vi "Accelerator_v2.001_small.vi"() -> ()   [LabVIEW 2013]
doc: "Acquire Accelerator Data"
uses:
  <instrlib>/niScope/Controls/niScope vertical coupling.ctl
  <instrlib>/niScope/Controls/niScope trigger slope.ctl
  <instrlib>/niScope/Controls/niScope trigger coupling.ctl
  <instrlib>/niScope/Controls/niScope trigger source.ctl
  Accelerator Measurement/Array_Defctl.ctl
  <vilib>/Utility/error.llb/DialogType.ctl
  <vilib>/Utility/miscctls.llb/LVPointTypeDef.ctl
  Public API/Dust_Event.ctl
  Public API/Signal.ctl
  Private/Role ID.ctl
  Private/Hardware ID.ctl
  Private/Estimate_source.ctl
  Functional Global Variables/Action Items.ctl
  <vilib>/Analysis/baseanly.llb/Mean (DBL).vi
  Private/PSU updated.vi
  <vilib>/addons/database/Connection.llb/Conn Execute.vi
  <vilib>/addons/database/Recordset.llb/Rec Fetch Recordset Data (R).vi
  <vilib>/addons/database/Recordset.llb/Rec Destroy - Connection.vi
  <instrlib>/niScope/Configure/Trigger/niScope Configure Trigger Edge.vi
  <instrlib>/niScope/Configure/Trigger/niScope Configure Trigger Immediate.vi
  <instrlib>/niScope/Acquire/Fetch/niScope Multi Fetch Cluster.vi
  <vilib>/addons/database/_DB Variant To Data/Database Variant To Data.xnode
  <vilib>/Analysis/NI_AALBase.lvlib
  <vilib>/addons/database/NI_Database_API.lvlib
panel:
  in  "Big Accelerator?":bool
  in  "Trigger":enum32{"Immediate", "Edge"}(tab)=enum."Edge"
  in  "Trigger Source Edge 2":T1="2" caption="Source"
  in  "Trigger Source Edge":T1="0" caption="Source"
  in  "Coupling":T2=1 items=["AC"=0, "DC"=1, "HF Reject"=3, "LF Reject"=4, "AC Plus HF Reject"=1001]
  in  "Slope":T3 caption="Trigger Slope"
  in  "Level":dbl=1.0 caption="Trigger Level" step=0.001 format="%.3f"
  in  "Delay":dbl caption="Trigger Delay" format="%.4p"
  in  "Reference Position (%)":dbl=40.0 caption="Ref Position" format="%.1f"
  in  "Bandwidth":dbl=-1.0 format="%.2f"
  in  "Vertical Coupling":T4=1 items=["AC", "DC", "Ground"]
  in  "Probe Attenuation":dbl=1.0 format="%.1f"
  in  "Vertical Offset":dbl format="%.4f"
  in  "Vertical Range":dbl=5.0 caption="Vertical Range (V)" format="%.2f"
  out "Actual Sample Rate":dbl=10000000.0 format="%.0p"
  in  "Min Record Length":i32=100000 caption="Min. Record Length"
  in  "Min Sample Rate":dbl=80000000.0 caption="Min. Sample Rate" step=1000000.0 format="%.2p"
  out "Actual Record Length":i32=100000
  out "Mass":dbl format="%#_3g"
  in  "Write to Database?":bool=TRUE
  in  "Limit":dbl
  in  "Limit Triggers":bool
  out "Acquisition #":i32
  in  "WFM Tag":string="trace"
  in  "Location":string="G:\\default"
  in  "Write Raw File?":bool
  out "Saving Raw File...":path=path "G:/2012_06_13_verify_timestamp_labview/trace00000"
  out "?":cluster{dbl, dbl}(knob)={0.0549, 2.0} scale=10.0..0.01
  in  "Ideal Time (Cursor)":dbl=2.0 step=0.01 format="%_2f"
  out "Time Between Triggers":dbl
  out "Average Frequency":dbl format="%#_4g"
  out "output cluster":T5
  out "error out 4":errorcluster
  out "error out 3":errorcluster
  out "# elements in queue":i32
  out "Stop condition":bool=TRUE
  out "created path":path=path "G:/default"
  out "Numeric":i32=92364
  out "error out 2":errorcluster
  out "Calibration":dbl=24700000000000.0
  out "Array":T6=["Dev1", "Dev2"]
  in  "Debug Mode\n(Confusing)":bool
  out "Multi Plot 2":cluster{dbl[], dbl[]}(graph) caption="Multi Plot"
  in  "Acceleration Voltage (MV)":dbl=2.0 format="%_2g"
  out "Charge":dbl format="%#_3g"
  out "Velocity (Est.)":dbl format="%#_6f"
  out "Final Detector (CH3)":waveform(dbl)(graph)={"t0"=timestamp(0 s since 1904-01-01), "dt"=1e-07, "Y"=[]}
  out "Charge Detector/PSU gate (CH2)":waveform(dbl)(graph)={"t0"=timestamp(0 s since 1904-01-01), "dt"=1e-07, "Y"=[]}
  out "Velocity Detectors (CH0 & CH1)":waveform(dbl)[](graph)
  in  "stop":bool=TRUE
  out "error out":errorcluster={"status"=FALSE, "code"=0, "source"="No Error"} {"code" format="%.0x"}
  # "File Parameters"
  # "Error Handling"
  # "Trigger"
  # "Channel"
  # "Vertical"
  # "Horizontal"
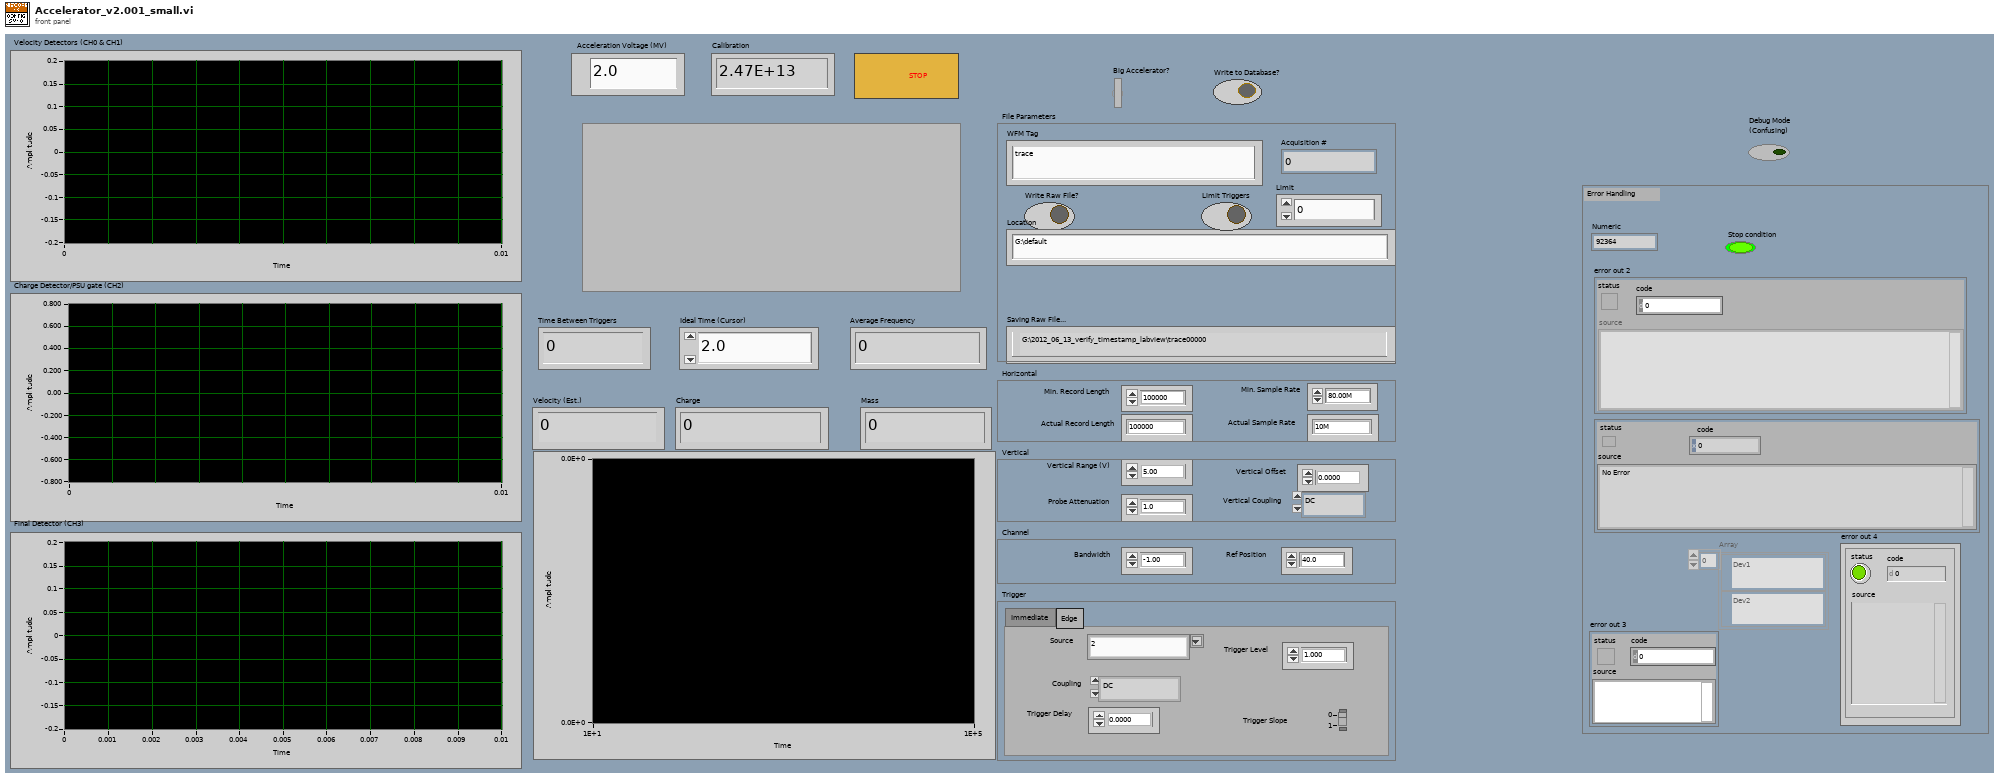
[diagram p1: front panel]
types:
  T1 = typedef "niScope trigger source.ctl" = string
  T2 = typedef "niScope trigger coupling.ctl" = u16
  T3 = typedef "niScope trigger slope.ctl" = i32
  T4 = typedef "niScope vertical coupling.ctl" = i32
  T5 = cluster{"File Path Control":path, "Array":waveform(dbl)[]}
  T6 = typedef "Array_Defctl.ctl" = refnum<k15>[]
  T7 = typedef "LVPointTypeDef.ctl" = cluster{"Horizontal":i16, "Vertical":i16}
  T8 = typedef "DialogType.ctl" = u16
  T9 = typedef "NI_Database_API.lvlib/Conn ObjectReference.ctl" = refnum<k1>
  T10 = typedef "NI_Database_API.lvlib/Rec ObjectReference.ctl" = refnum<k1>
  T11 = cluster{"Integer Timestamp":dbl, "Max Velocity":dbl, "Min Velocity":dbl}
  T12 = cluster{"first point time":dbl, "xIncrement":dbl, "Waveforms":dbl[]}[]
  T13 = typedef "Dust_Event.ctl" = cluster{"Time Stamp":timestamp, "Velocity":sgl, "Mass":sgl, "Charge":sgl, "Radius":sgl, "Array":T14[], "Dust Event ID":i64, "Passed_3rd_Detector":bool, "Estimate Source":T17, "Estimate Quality":sgl}
  T14 = typedef "Signal.ctl" = cluster{"Signal ID":i64, "Time Stamp":timestamp, "Dust Event ID":i64, "Role ID":T15, "Data":sgl[], "Signal Length":i32, "dt":sgl, "Offset":dbl, "Hardware ID":T16}
  T15 = typedef "Role ID.ctl" = enum16{"First_Detector", "Second_Detector", "Third_Detector", "LeCroy_CH1", "LeCroy_CH2", "LeCroy_CH3", "LeCroy_CH4", "PSU"}
  T16 = typedef "Hardware ID.ctl" = enum16{"Unknown", "CSA 1", "CSA 2", "CSA 3", "CSA 4", "CSA 5", "CSA 6"}
  T17 = typedef "Estimate_source.ctl" = i8
  T18 = typedef "Action Items.ctl" = enum16{"Initialize", "Get", "Set"}
  T19 = cluster{"relativeInitialX":dbl, "xIncrement":dbl, "wfm":dbl[]}[]
  T20 = cluster{"first point time":dbl, "xIncrement":dbl, "Waveforms":dbl[]}
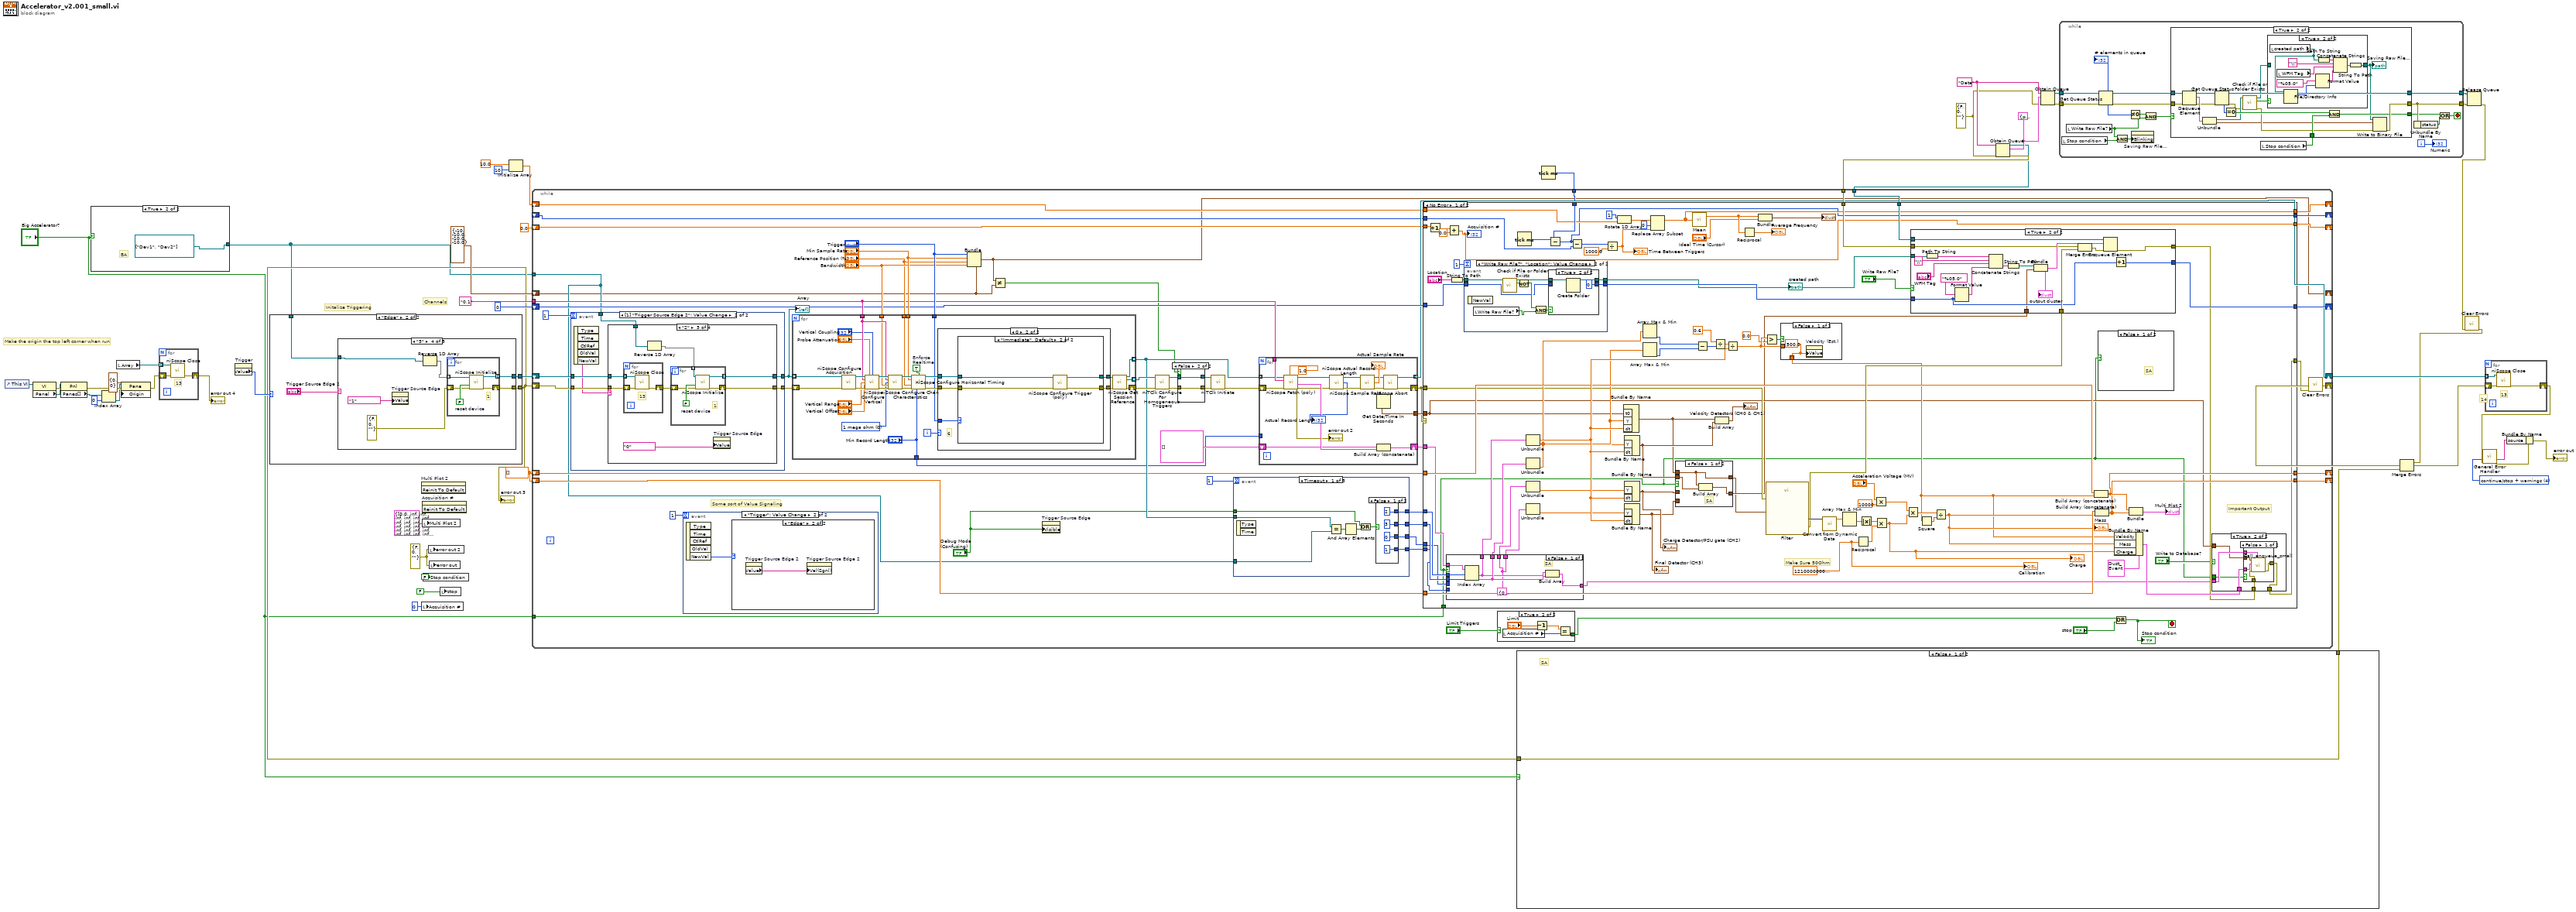
[diagram p0: block diagram]
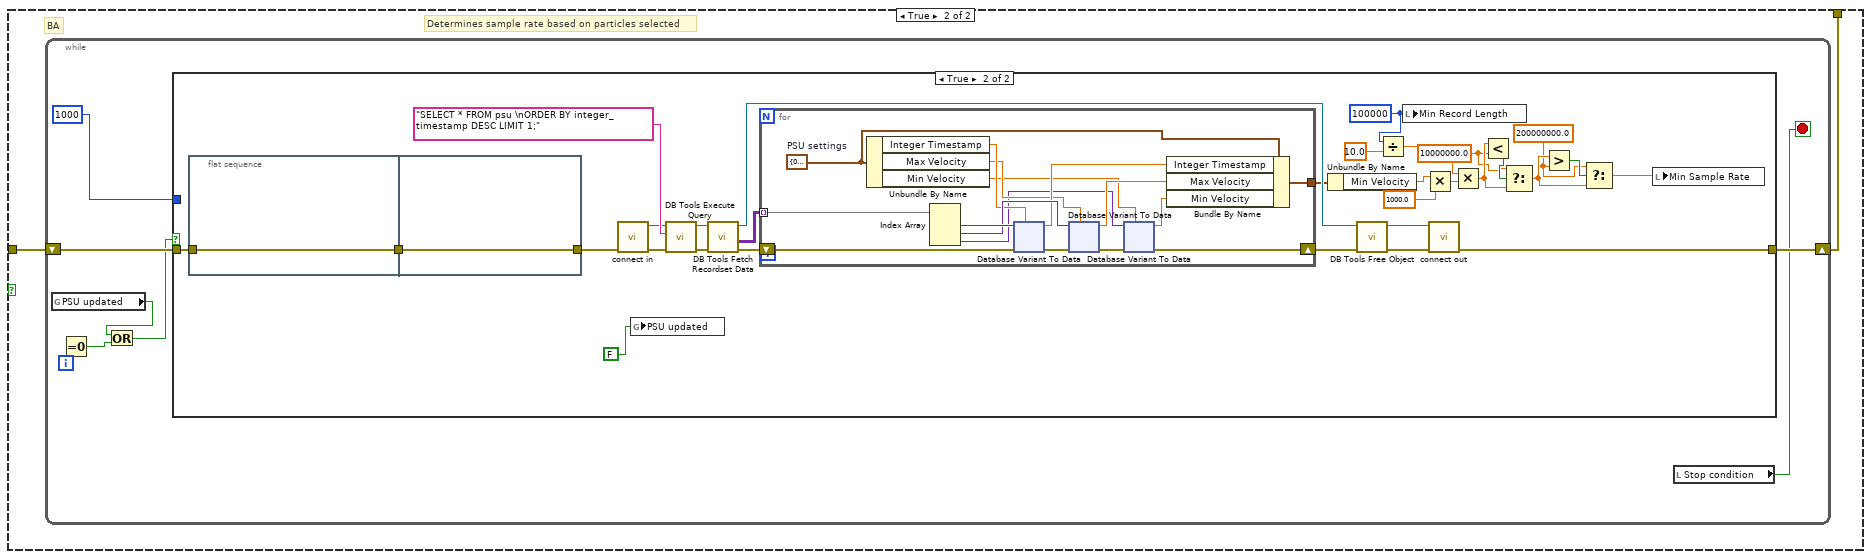
[diagram p2: hidden frame]
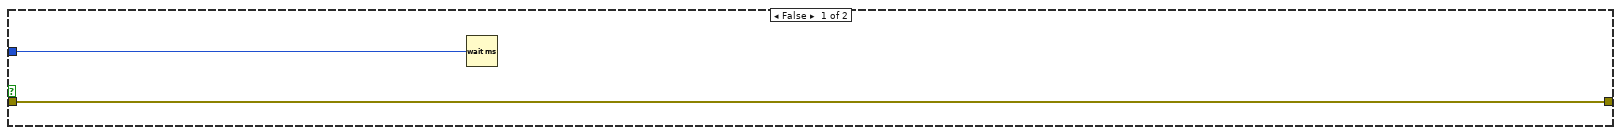
[diagram p3: hidden frame]
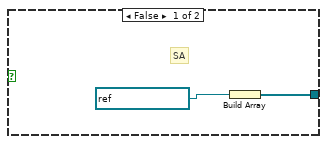
[diagram p4: hidden frame]
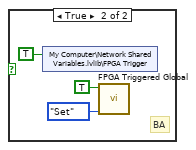
[diagram p5: hidden frame]
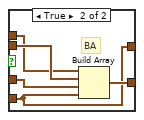
[diagram p6: hidden frame]
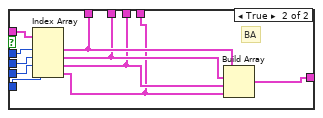
[diagram p7: hidden frame]
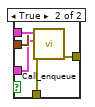
[diagram p9: hidden frame]
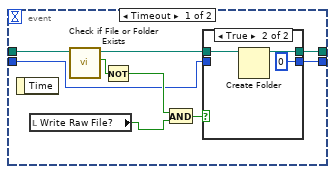
[diagram p10: hidden frame]
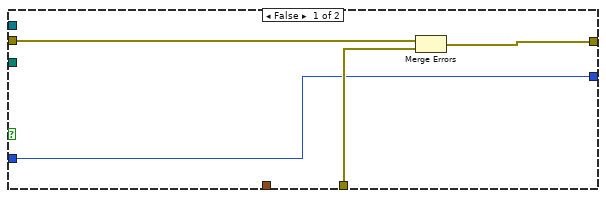
[diagram p13: hidden frame]
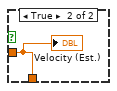
[diagram p14: hidden frame]
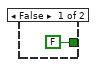
[diagram p16: hidden frame]
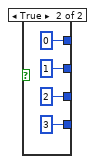
[diagram p17: hidden frame]
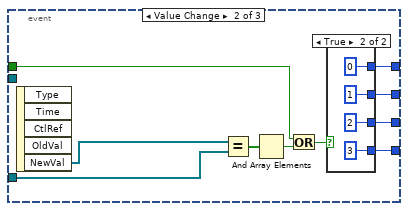
[diagram p18: hidden frame]
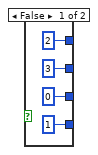
[diagram p19: hidden frame]
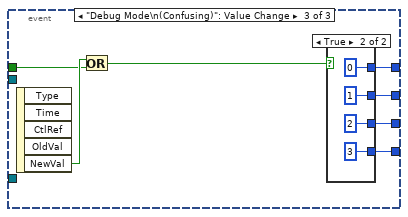
[diagram p20: hidden frame]
diagram:
  w15 = dbl[] []
  w22 = errorcluster {"status"=FALSE, "code"=0, "source"=""} ("error out")
  w27 = errorcluster {"status"=FALSE, "code"=0, "source"=""} ("error out")
  w28 = cluster{path, waveform(sgl)[]} {path "", []} ("output cluster")
  w29 = "Data" ("name (unnamed)")
  w20 = T8 4 items=["no dialog", "OK message", "continue or stop message", "OK message + warnings", "continue/stop + warnings"] ("type of dialog (OK msg:1)")
  # "Channels"
  # "Make the origin the top left corner when run"
  # "Initalize Triggering"
  # "14"
  n1 = control-ref of="This VI"() -> (w11:refnum<vi>)
  n2 = property class="VI"(reference=w11) -> (error out=w10:errorcluster, "Panel"=w9:refnum<vi>)  [unwired: 1 in, 1 out]
  n3 = property class="Pnl"(reference=w9, error in=w10) -> (error out=w8:errorcluster, "Panes[]"=w7:refnum<vi>[])  [unwired: 1 out]
  n4 = case shown="True" "Big Accelerator?" {
    tunnel: [w51 refnum<k15>[] ["Dev1", "Dev2"] ("Resources")] -> w2
    frame False {
      # "SA"
      n5 = Build Array(refnum<k15> "Dev1" ("resource name")) -> (w51:refnum<k15>[])
    }
    frame True {
      # "BA"
    }
  }
  n6 = Index Array(array=w7, index=0) -> (element=w5:refnum<vi>)
  n7 = local read "Array"() -> (w30:T6)
  n8 = property class="Pane"(reference=w5, error in=w8, "Origin"=T7 {"Horizontal"=0, "Vertical"=0}) -> (error out=w3:errorcluster)  [unwired: 1 out]
  n9 = for {
    tunnel: w30 -> [w54] mode=indexing
    shift-right: [w56] -> w25
    shift-left: w3 -> [w55]
    # "13"
    n10 = call <instrlib>:"niScope Close.vi"("instrument handle"=w54, "error in"=w55) -> ("error out"=w56:errorcluster)  [unwired: 13 in]
  }
  "error out 4" <- w25
  n11 = property on="Trigger" class="TabCtl (strict)"() -> ("Value"=w39:enum32{"Immediate", "Edge"})  [unwired: 2 in, 2 out]
  n12 = case shown="\"Edge\"" w39 {
    tunnel: [w59 w69] -> w49
    tunnel: [w58 w68] -> w13
    tunnel: w2 -> [w57 w66]
    frame "Immediate", Default {
      n13 = for {
        tunnel: w57 -> [w64] mode=indexing
        tunnel: [w62] -> w59 mode=indexing
        shift-right: [w61] -> w58
        shift-left: errorcluster {"status"=FALSE, "code"=0, "source"=""} ("error out") -> [w63]
        w65 = FALSE  # reset device
        n14 = call <instrlib>:"niScope Initialize.vi"("resource name"=w64, "reset device"=w65, "error in"=w63) -> ("instrument handle"=w62:refnum<k15>, "error out"=w61:errorcluster)  [unwired: 11 in]
      }
    }
    frame "Edge" {
      n15 = case shown="\"3\"" "Trigger Source Edge 2" {
        tunnel: [w74 w83 w94 w105 w116] -> w69
        tunnel: [w73 w82 w93 w104 w115] -> w68
        tunnel: w66 -> [w70 w80 w90 w101 w112]
        frame "0", Default {
          n16 = property on="Trigger Source Edge" class="CmbBox (strict)"("Value"=T1 "0" ("Trigger Source Edge")) -> ()  [unwired: 2 in, 2 out]
          n17 = for {
            tunnel: w70 -> [w78] mode=indexing
            tunnel: [w76] -> w74 mode=indexing
            shift-right: [w75] -> w73
            shift-left: errorcluster {"status"=FALSE, "code"=0, "source"=""} ("error out") -> [w77]
            w79 = FALSE  # reset device
            n18 = call <instrlib>:"niScope Initialize.vi"("resource name"=w78, "reset device"=w79, "error in"=w77) -> ("instrument handle"=w76:refnum<k15>, "error out"=w75:errorcluster)  [unwired: 11 in]
          }
        }
        frame "1" {
          n19 = property on="Trigger Source Edge" class="CmbBox (strict)"("Value"=T1 "1" ("Trigger Source Edge")) -> ()  [unwired: 2 in, 2 out]
          n20 = for {
            tunnel: w80 -> [w88] mode=indexing
            tunnel: [w86] -> w83 mode=indexing
            shift-right: [w85] -> w82
            shift-left: errorcluster {"status"=FALSE, "code"=0, "source"=""} ("error out") -> [w87]
            w89 = FALSE  # reset device
            # "1"
            n21 = call <instrlib>:"niScope Initialize.vi"("resource name"=w88, "reset device"=w89, "error in"=w87) -> ("instrument handle"=w86:refnum<k15>, "error out"=w85:errorcluster)  [unwired: 11 in]
          }
        }
        frame "2" {
          n22 = property on="Trigger Source Edge" class="CmbBox (strict)"("Value"=T1 "0" ("Trigger Source Edge")) -> ()  [unwired: 2 in, 2 out]
          n23 = Reverse 1D Array(array=w90) -> (reversed array=w91:refnum<k15>[])
          n24 = for {
            tunnel: w91 -> [w99] mode=indexing
            tunnel: [w97] -> w94 mode=indexing
            shift-right: [w96] -> w93
            shift-left: errorcluster {"status"=FALSE, "code"=0, "source"=""} ("error out") -> [w98]
            w100 = FALSE  # reset device
            # "1"
            n25 = call <instrlib>:"niScope Initialize.vi"("resource name"=w99, "reset device"=w100, "error in"=w98) -> ("instrument handle"=w97:refnum<k15>, "error out"=w96:errorcluster)  [unwired: 11 in]
          }
        }
        frame "3" {
          n26 = property on="Trigger Source Edge" class="CmbBox (strict)"("Value"=T1 "1" ("Trigger Source Edge")) -> ()  [unwired: 2 in, 2 out]
          n27 = Reverse 1D Array(array=w101) -> (reversed array=w102:refnum<k15>[])
          n28 = for {
            tunnel: w102 -> [w110] mode=indexing
            tunnel: [w108] -> w105 mode=indexing
            shift-right: [w107] -> w104
            shift-left: errorcluster {"status"=FALSE, "code"=0, "source"=""} ("error out") -> [w109]
            w111 = FALSE  # reset device
            # "1"
            n29 = call <instrlib>:"niScope Initialize.vi"("resource name"=w110, "reset device"=w111, "error in"=w109) -> ("instrument handle"=w108:refnum<k15>, "error out"=w107:errorcluster)  [unwired: 11 in]
          }
        }
        frame "VAL_EXTERNAL" {
          n30 = property on="Trigger Source Edge" class="CmbBox (strict)"("Value"=T1 "VAL_EXTERNAL" ("Trigger Source Edge")) -> ()  [unwired: 2 in, 2 out]
          n31 = for {
            tunnel: w112 -> [w120] mode=indexing
            tunnel: [w118] -> w116 mode=indexing
            shift-right: [w117] -> w115
            shift-left: errorcluster {"status"=FALSE, "code"=0, "source"=""} ("error out") -> [w119]
            w121 = FALSE  # reset device
            n32 = call <instrlib>:"niScope Initialize.vi"("resource name"=w120, "reset device"=w121, "error in"=w119) -> ("instrument handle"=w118:refnum<k15>, "error out"=w117:errorcluster)  [unwired: 11 in]
          }
        }
      }
    }
  }
  "error out 3" <- w13
  n33 = invoke on="Multi Plot 2" class="XYGraph (strict)" method="Reinit To Default"() -> ()  [unwired: 3 in, 3 out]
  n34 = local write "Acquisition #"(0 ("Acquisition #")) -> ()
  n35 = invoke on="Acquisition #" class="DigNum (strict)" method="Reinit To Default"() -> ()  [unwired: 3 in, 3 out]
  n36 = local write "Multi Plot 2"(cluster{dbl[], dbl[]} {[0.0, inf, inf, inf, inf, inf, inf, inf, inf, inf, inf, inf, inf, inf, inf, inf, inf, inf, inf, inf, inf, inf, inf, inf, inf, inf, inf, inf, inf, inf, inf, inf, inf, inf, inf, inf, inf, inf, inf, inf, inf], [0.0, 0.0, 0.0, 0.0, 0.0, 0.0, 0.0, 0.0, 0.0, 0.0, 0.0, 0.0, 0.0, 0.0, 0.0, 0.0, 0.0, 0.0, 0.0, 0.0, 0.0, 0.0, 0.0, 0.0, 0.0, 0.0, 0.0, 0.0, 0.0, 0.0, 0.0, 0.0, 0.0, 0.0, 0.0, 0.0, 0.0, 0.0, 0.0, 0.0, 0.0]} ("Multi Plot 2")) -> ()
  n37 = local write "Stop condition"(FALSE ("x .or. y?")) -> ()
  n38 = local write "error out 2"(w22) -> ()
  n39 = local write "error out"(w22) -> ()
  n40 = local write "stop"(FALSE ("stop")) -> ()
  n41 = Initialize Array(10.0 ("element"), 10 ("dimension size")) -> (w41:dbl[])
  n42 = case shown="False" "Big Accelerator?" {
    tunnel: w13 -> [w122 w124]
    tunnel: [w122 w123] -> w12
    frame False {
      # "SA"
    }
    frame True {
      # "BA"
      # "Determines sample rate based on particles selected"
      n43 = while {
        shift-right: [w131] -> w123
        shift-left: w124 -> [w132]
        i -> [w130]
        stop <- w129 stop-if-true
        n44 = global read "PSU updated.vi" "PSU updated"() -> (w128:bool)
        n45 = Equal To 0?(x=w130) -> (x = 0?=w126:bool)
        n46 = Or(x=w128, y=w126) -> (x .or. y?=w127:bool)
        n47 = case shown="True" w127 {
          tunnel: w132 -> [w133 w163]
          tunnel: [w133 w162] -> w131
          tunnel: 1000 -> [w134 _]
          frame False {
            n48 = Wait (ms)(milliseconds to wait=w134) -> ()  [unwired: 1 out]
          }
          frame True {
            w136 = 200000000.0 ("y")
            w139 = 10000000.0 ("y")
            w146 = 100000 ("Min Record Length")
            n49 = flat-sequence {
              tunnel: [w165] -> w164
              tunnel: w163 -> [w165]
              tunnel: w164 -> [w166]
              tunnel: [w166] -> w149
              frame #0 {
              }
              frame #1 {
              }
            }
            n50 = call "connect in.vi"("error in (no error)"=w149) -> ("error out"=w153:errorcluster, "Database Connection"=w152:T9)  [unwired: 6 in, 1 out]
            n51 = global write "PSU updated.vi" "PSU updated"(FALSE ("PSU updated")) -> ()
            n52 = call-poly <vilib>:"DB Tools Execute Query.vi"("error in (no error)"=w153, "SQL query"="SELECT * FROM psu \nORDER BY integer_timestamp DESC LIMIT 1;", "connection reference"=w152) -> ("error out"=w155:errorcluster, "recordset reference"=w154:T10)  [unwired: 5 in]
            n53 = call-poly <vilib>:"DB Tools Fetch Recordset Data.vi"("error in (no error)"=w155, "recordset reference"=w154) -> ("error out"=w161:errorcluster, "recordset data"=w160:variant[][], "recordset reference out"=w156:T10)  [unwired: 3 in]
            n54 = for {
              tunnel: w160 -> [w182] mode=indexing
              shift-right: [w167] -> w150
              shift-left: w161 -> [w178]
              tunnel: [w177] -> w151
              w172 = T11 {"Integer Timestamp"=0.0, "Max Velocity"=0.0, "Min Velocity"=0.0}  # PSU settings
              n55 = Unbundle By Name(w172) -> ("Integer Timestamp"=w176:dbl, "Max Velocity"=w173:dbl, "Min Velocity"=w170:dbl)
              n56 = Index Array(array=w182) -> (element #1=w181:variant, element #2=w180:variant, element #3=w171:variant)  [unwired: 3 in]
              n57 = xnode "Database Variant To Data"("database variant"=w181, "error in"=w178, "type"=w176) -> ("data"=w175:dbl, "error out"=w179:errorcluster)
              n58 = xnode "Database Variant To Data"("database variant"=w180, "error in"=w179, "type"=w173) -> ("data"=w174:dbl, "error out"=w168:errorcluster)
              n59 = xnode "Database Variant To Data"("database variant"=w171, "error in"=w168, "type"=w170) -> ("data"=w169:dbl, "error out"=w167:errorcluster)
              n60 = Bundle By Name(cluster=w172, "Integer Timestamp"=w175, "Max Velocity"=w174, "Min Velocity"=w169) -> (w177:T11)
            }
            n61 = Unbundle By Name(w151) -> ("Min Velocity"=w145:dbl)
            n62 = call-poly <vilib>:"DB Tools Free Object.vi"("error in (no error)"=w150, "recordset reference"=w156) -> ("error out"=w157:errorcluster, "connection reference"=w158:T9)  [unwired: 8 in]
            n63 = Divide(x=w146, y=10.0) -> (x/y=w142:dbl)
            n64 = local write "Min Record Length"(w146) -> ()
            n65 = Multiply(x=w145, y=1000.0) -> (x*y=w143:dbl)
            n66 = call "connect out.vi"("error in (no error)"=w157, "connection reference"=w158) -> ("error out"=w162:errorcluster)  [unwired: 9 in]
            n67 = Multiply(x=w142, y=w143) -> (x*y=w140:dbl)
            n68 = Less?(x=w140, y=w139) -> (x < y?=w141:bool)
            n69 = Select(t=w139, s=w141, f=w140) -> (s? t:f=w138:dbl)
            n70 = Greater?(x=w138, y=w136) -> (0:w137:bool)
            n71 = Select(t=w136, s=w137, f=w138) -> (s? t:f=w135:dbl)
            n72 = local write "Min Sample Rate"(w135) -> ()
          }
        }
        n73 = local read "Stop condition"() -> (w129:bool)
      }
    }
  }
  n74 = Tick Count (ms)() -> (millisecond timer value=w44:u32)
  n75 = Obtain Queue(name (unnamed)=w29, element data type=w28, error in (no error)=w27) -> (queue out=w24:refnum<queue>, error out=w37:errorcluster)  [unwired: 2 in, 1 out]
  n76 = while {
    shift-right: [w291] -> w23
    shift-left: w13 -> [w296]
    shift-right: [w280] -> _
    shift-left: cluster{i32, dbl, dbl, dbl} {-10, -10.0, -10.0, -10.0} -> [w281]
    tunnel: w44 -> [w288]
    shift-right: [w286] -> _
    shift-left: w41 -> [w287]
    shift-right: [w285] -> _
    shift-left: _ -> [w289]
    shift-right: [w323] -> _
    shift-left: w15 -> [w300]
    shift-right: [w322] -> _
    shift-left: w15 -> [w321]
    tunnel: "0,1" ("Channel Name") -> [w320]
    shift-right: [w297] -> w38
    shift-left: w49 -> [w318]
    tunnel: w24 -> [w307]
    tunnel: w37 -> [w306]
    shift-right: [w305] -> _
    shift-left: 0 -> [w304]
    shift-right: [w283] -> _
    shift-left: 0.0 -> [w284]
    tunnel: w2 -> [w282]
    tunnel: "Big Accelerator?" -> [w279]
    stop <- w295 stop-if-true
    # "Some sort of Value Signaling"
    n77 = event shown="[1] \"Trigger Source Edge 2\": Value Change" {
      selector: _ -> [_ _]
      dyn-events: _ -> [_ _]
      timeout: 1 -> [_ _]
      tunnel: w318 -> [w604 w609]
      tunnel: [w604 w607] -> w315
      tunnel: w296 -> [w603 w610]
      tunnel: [w603 w606] -> w316
      tunnel: w282 -> [_ w605]
      event Timeout {
        n78 = event-data() -> ()  [unwired: 1 in, 2 out]
      }
      event Value Change {
        n79 = event-data() -> ("NewVal"=w608:T1)  [unwired: 1 in, 4 out]
        n80 = case shown="\"2\"" w608 {
          selector: w608 -> [w612 w627 _ _]
          tunnel: w609 -> [w614 w629 w647 w661]
          tunnel: [w616 w631 w645 w662] -> w607
          tunnel: w610 -> [w613 w628 w646 w660]
          tunnel: [w615 w630 w644 w663] -> w606
          tunnel: w605 -> [w611 w626 w641 w658]
          frame "0", Default {
            n81 = for {
              tunnel: w614 -> [w618] mode=indexing
              shift-right: [w620] -> w617
              shift-left: w613 -> [w619]
              # "13"
              n82 = call <instrlib>:"niScope Close.vi"("instrument handle"=w618, "error in"=w619) -> ("error out"=w620:errorcluster)  [unwired: 13 in]
            }
            n83 = for {
              tunnel: [w624] -> w616 mode=indexing
              shift-right: [w623] -> w615
              shift-left: w617 -> [w621]
              tunnel: w611 -> [w622] mode=indexing
              w625 = FALSE  # reset device
              # "1"
              n84 = call <instrlib>:"niScope Initialize.vi"("resource name"=w622, "reset device"=w625, "error in"=w621) -> ("instrument handle"=w624:refnum<k15>, "error out"=w623:errorcluster)  [unwired: 11 in]
            }
            n85 = property on="Trigger Source Edge" class="CmbBox (strict)"("Value"=w612) -> ()  [unwired: 2 in, 2 out]
          }
          frame "1" {
            n86 = for {
              tunnel: w629 -> [w633] mode=indexing
              shift-right: [w635] -> w632
              shift-left: w628 -> [w634]
              # "13"
              n87 = call <instrlib>:"niScope Close.vi"("instrument handle"=w633, "error in"=w634) -> ("error out"=w635:errorcluster)  [unwired: 13 in]
            }
            n88 = for {
              tunnel: [w639] -> w631 mode=indexing
              shift-right: [w638] -> w630
              shift-left: w632 -> [w636]
              tunnel: w626 -> [w637] mode=indexing
              w640 = FALSE  # reset device
              # "1"
              n89 = call <instrlib>:"niScope Initialize.vi"("resource name"=w637, "reset device"=w640, "error in"=w636) -> ("instrument handle"=w639:refnum<k15>, "error out"=w638:errorcluster)  [unwired: 11 in]
            }
            n90 = property on="Trigger Source Edge" class="CmbBox (strict)"("Value"=w627) -> ()  [unwired: 2 in, 2 out]
          }
          frame "2" {
            n91 = for {
              tunnel: w647 -> [w649] mode=indexing
              shift-right: [w651] -> w648
              shift-left: w646 -> [w650]
              # "13"
              n92 = call <instrlib>:"niScope Close.vi"("instrument handle"=w649, "error in"=w650) -> ("error out"=w651:errorcluster)  [unwired: 13 in]
            }
            n93 = Reverse 1D Array(array=w641) -> (reversed array=w642:refnum<k15>[])
            n94 = for {
              tunnel: [w655] -> w645 mode=indexing
              shift-right: [w654] -> w644
              shift-left: w648 -> [w652]
              tunnel: w642 -> [w653] mode=indexing
              w656 = FALSE  # reset device
              # "1"
              n95 = call <instrlib>:"niScope Initialize.vi"("resource name"=w653, "reset device"=w656, "error in"=w652) -> ("instrument handle"=w655:refnum<k15>, "error out"=w654:errorcluster)  [unwired: 11 in]
            }
            n96 = property on="Trigger Source Edge" class="CmbBox (strict)"("Value"=T1 "0" ("Trigger Source Edge")) -> ()  [unwired: 2 in, 2 out]
          }
          frame "3" {
            n97 = for {
              tunnel: w661 -> [w665] mode=indexing
              shift-right: [w667] -> w664
              shift-left: w660 -> [w666]
              # "13"
              n98 = call <instrlib>:"niScope Close.vi"("instrument handle"=w665, "error in"=w666) -> ("error out"=w667:errorcluster)  [unwired: 13 in]
            }
            n99 = Reverse 1D Array(array=w658) -> (reversed array=w657:refnum<k15>[])
            n100 = for {
              tunnel: [w671] -> w662 mode=indexing
              shift-right: [w670] -> w663
              shift-left: w664 -> [w668]
              tunnel: w657 -> [w669] mode=indexing
              w672 = FALSE  # reset device
              # "1"
              n101 = call <instrlib>:"niScope Initialize.vi"("resource name"=w669, "reset device"=w672, "error in"=w668) -> ("instrument handle"=w671:refnum<k15>, "error out"=w670:errorcluster)  [unwired: 11 in]
            }
            n102 = property on="Trigger Source Edge" class="CmbBox (strict)"("Value"=T1 "1" ("Trigger Source Edge")) -> ()  [unwired: 2 in, 2 out]
          }
        }
      }
    }
    "Array" <- w315
    n103 = event shown="[1] \"Trigger\": Value Change" {
      selector: _ -> [_ _]
      dyn-events: _ -> [_ _]
      timeout: 1 -> [_ _]
      event Timeout {
        n104 = event-data() -> ()  [unwired: 1 in, 2 out]
      }
      event "Trigger": Value Change {
        n105 = event-data() -> ("NewVal"=w601:enum32{"Immediate", "Edge"})  [unwired: 1 in, 4 out]
        n106 = case shown="\"Edge\"" w601 {
          frame "Immediate", Default {
          }
          frame "Edge" {
            n107 = property on="Trigger Source Edge 2" class="CmbBox (strict)"() -> ("Value"=w602:T1)  [unwired: 2 in, 2 out]
            n108 = property on="Trigger Source Edge 2" class="CmbBox (strict)"("Val(Sgnl)"=w602) -> ()  [unwired: 2 in, 2 out]
          }
        }
      }
    }
    n109 = for {
      tunnel: w315 -> [w706] mode=indexing
      shift-right: [w684] -> w327
      shift-left: w316 -> [w705]
      tunnel: w320 -> [w697]
      tunnel: "Min Sample Rate" -> [w690]
      tunnel: "Trigger" -> [w689]
      tunnel: "Bandwidth" -> [w687]
      tunnel: "Reference Position (%)" -> [w686]
      tunnel: [w683] -> w309 mode=indexing
      tunnel: [w682] -> w324 mode=indexing
      tunnel: ["Min Record Length"] -> w308
      i -> [w691]
      w679 = u32 0 items=["1 mega ohm"] ("input impedance")
      w704 = TRUE  # Enforce Realtime
      n110 = call <instrlib>:"niScope Configure Acquisition.vi"("instrument handle"=w706, "error in"=w705) -> ("instrument handle out"=w702:refnum<k15>, "error out"=w703:errorcluster)  [unwired: 12 in]
      n111 = call <instrlib>:"niScope Configure Vertical.vi"("instrument handle"=w702, "probe attenuation"="Probe Attenuation", "vertical coupling"="Vertical Coupling", "channels"=w697, "vertical range"="Vertical Range", "vertical offset"="Vertical Offset", "error in"=w703) -> ("instrument handle out"=w701:refnum<k15>, "error out"=w700:errorcluster)  [unwired: 7 in]
      n112 = call <instrlib>:"niScope Configure Chan Characteristics.vi"("instrument handle"=w701, "channels"=w697, "input impedance"=w679, "maximum input frequency"=w687, "error in"=w700) -> ("instrument handle out"=w698:refnum<k15>, "error out"=w699:errorcluster)  [unwired: 9 in]
      n113 = call <instrlib>:"niScope Configure Horizontal Timing.vi"("instrument handle"=w698, "enforce realtime"=w704, "min sample rate"=w690, "reference position"=w686, "error in"=w699, "min record length"="Min Record Length") -> ("instrument handle out"=w693:refnum<k15>, "error out"=w694:errorcluster)  [unwired: 8 in]
      n114 = case shown="0" w691 {
        tunnel: w694 -> [w707 w713]
        tunnel: w693 -> [w708 w712]
        tunnel: [w708 w711] -> w681
        tunnel: [w707 w710] -> w685
        tunnel: w689 -> [_ w709]
        frame 1, Default {
        }
        frame 0 {
          # "6"
          n115 = case "Trigger Selection" shown="\"Immediate\", Default" w709 {
            tunnel: w713 -> [w722 w726]
            tunnel: [w719 w723] -> w710
            tunnel: w712 -> [w721 w725]
            tunnel: [w720 w724] -> w711
            frame "Edge" {
              n116 = call-poly <instrlib>:"niScope Configure Trigger (poly).vi"("instrument handle"=w721, "trigger slope"="Slope", "trigger coupling"="Coupling", "trigger source"="Trigger Source Edge", "trigger level"="Level", "error in"=w722, "trigger delay"="Delay") -> ("instrument handle out"=w720:refnum<k15>, "error out"=w719:errorcluster)  [unwired: 7 in]
            }
            frame "Immediate", Default {
              n117 = call-poly <instrlib>:"niScope Configure Trigger (poly).vi"("instrument handle"=w725, "error in"=w726) -> ("instrument handle out"=w724:refnum<k15>, "error out"=w723:errorcluster)  [unwired: 12 in]
            }
          }
        }
      }
      n118 = call <instrlib>:"niScope Get Session Reference.vi"("instrument handle"=w681, "error in"=w685) -> ("instrument handle out"=w683:refnum<k15>, "session reference"=w682:refnum<k20>, "error out"=w684:errorcluster)  [unwired: 11 in]
    }
    n119 = Bundle(cluster=w281, "Trigger", "Min Sample Rate", "Reference Position (%)", "Bandwidth") -> (w280:cluster{i32, dbl, dbl, dbl})
    n120 = Not Equal?(x=w280, y=w281) -> (x != y?=w298:bool)
    n121 = property on="Trigger Source Edge" class="CmbBox (strict)"("Visible"="Debug Mode\n(Confusing)") -> ()  [unwired: 2 in, 2 out]
    n122 = call <instrlib>:"niTClk Configure For Homogeneous Triggers.vi"("error in (no error)"=w327, "sessions"=w324) -> ("error out"=w326:errorcluster, "sessions out"=w325:refnum<k20>[])  [unwired: 8 in]
    n123 = case shown="False" w298 {
      tunnel: [w676 w678] -> w334
      tunnel: [w675 w677] -> w333
      tunnel: w325 -> [w673 w678]
      tunnel: w326 -> [w674 w677]
      frame True {
        n124 = call <instrlib>:"niTClk Synchronize.vi"("error in (no error)"=w674, "sessions"=w673) -> ("error out"=w675:errorcluster, "sessions out"=w676:refnum<k20>[])  [unwired: 8 in]
      }
      frame False {
      }
    }
    n125 = call <instrlib>:"niTClk Initiate.vi"("error in (no error)"=w333, "sessions"=w334) -> ("error out"=w335:errorcluster)  [unwired: 8 in, 1 out]
    n126 = event shown="[0] Timeout" {
      selector: _ -> [_ _ _]
      dyn-events: _ -> [_ _ _]
      timeout: 1 -> [_ _ _]
      tunnel: [w559 w576 w592] -> w314
      tunnel: [w558 w575 w591] -> w313
      tunnel: [w557 w574 w590] -> w312
      tunnel: [w556 w573 w589] -> w311
      tunnel: w309 -> [w555 _ _]
      tunnel: "Debug Mode\n(Confusing)" -> [w551 w572 w586]
      tunnel: w282 -> [w550 w568 _]
      event Timeout {
        n127 = event-data() -> ()  [unwired: 1 in, 2 out]
        n128 = Equal?(x=w555, y=w550) -> (x = y?=w554:bool[])
        n129 = And Array Elements(Boolean array=w554) -> (logical AND=w552:bool)
        n130 = Or(x=w551, y=w552) -> (x .or. y?=w553:bool)
        n131 = case shown="False" w553 {
          tunnel: [2 ("index") 0 ("index")] -> w559
          tunnel: [3 ("index") 1 ("index")] -> w558
          tunnel: [0 ("index") 2 ("index")] -> w557
          tunnel: [1 ("index") 3 ("index")] -> w556
          frame False {
          }
          frame True {
          }
        }
      }
      event Value Change {
        n132 = event-data() -> ("NewVal"=w569:T6)  [unwired: 1 in, 4 out]
        n133 = Equal?(x=w569, y=w568) -> (x = y?=w577:bool[])
        n134 = And Array Elements(Boolean array=w577) -> (logical AND=w571:bool)
        n135 = Or(x=w572, y=w571) -> (x .or. y?=w570:bool)
        n136 = case shown="True" w570 {
          tunnel: [2 ("index") 0 ("index")] -> w576
          tunnel: [3 ("index") 1 ("index")] -> w575
          tunnel: [0 ("index") 2 ("index")] -> w574
          tunnel: [1 ("index") 3 ("index")] -> w573
          frame False {
          }
          frame True {
          }
        }
      }
      event "Debug Mode\n(Confusing)": Value Change {
        n137 = event-data() -> ("NewVal"=w587:bool)  [unwired: 1 in, 4 out]
        n138 = Or(x=w587, y=w586) -> (x .or. y?=w588:bool)
        n139 = case shown="True" w588 {
          tunnel: [2 ("index") 0 ("index")] -> w592
          tunnel: [3 ("index") 1 ("index")] -> w591
          tunnel: [0 ("index") 2 ("index")] -> w590
          tunnel: [1 ("index") 3 ("index")] -> w589
          frame False {
          }
          frame True {
          }
        }
      }
    }
    n140 = for {
      tunnel: w320 -> [w545]
      tunnel: w309 -> [w541] mode=indexing
      shift-right: [w549] -> w299
      shift-left: T12 [] ("Waveform Graph") -> [w543]
      shift-right: [w532] -> w292
      shift-left: w335 -> [w542]
      tunnel: w308 -> [_]
      tunnel: [w534] -> w297 mode=indexing
      tunnel: [w540] -> w301
      n141 = call-poly <instrlib>:"niScope Fetch (poly).vi"("timeout"=1.0 ("Timeout (s)"), "error in"=w542, "channels"=w545, "instrument handle"=w541) -> ("error out"=w536:errorcluster, "waveform"=w544:T19, "instrument handle out"=w537:refnum<k15>)  [unwired: 4 in, 1 out]
      "error out 2" <- w536
      n142 = call <instrlib>:"niScope Actual Record Length.vi"("instrument handle"=w537, "error in"=w536) -> ("instrument handle out"=w548:refnum<k15>, "actual record length"=→"Actual Record Length":i32, "error out"=w547:errorcluster)  [unwired: 11 in]
      n143 = call <instrlib>:"niScope Sample Rate.vi"("instrument handle"=w548, "error in"=w547) -> ("instrument handle out"=w535:refnum<k15>, "actual sample rate"=→"Actual Sample Rate":dbl, "error out"=w533:errorcluster)  [unwired: 11 in]
      n144 = Get Date/Time In Seconds() -> (seconds since 1Jan1904=w540:timestamp)
      n145 = Build Array (concatenate)(w543, w544) -> (w549:T19)
      n146 = call <instrlib>:"niScope Abort.vi"("instrument handle"=w535, "error in"=w533) -> ("instrument handle out"=w534:refnum<k15>, "error out"=w532:errorcluster)  [unwired: 12 in]
    }
    n147 = case shown="No Error" w292 {
      tunnel: [w409 w524] -> w323
      tunnel: [w408 w525] -> w322
      tunnel: w321 -> [w407 w525]
      tunnel: w314 -> [w351 _]
      tunnel: w313 -> [w350 _]
      tunnel: w312 -> [w349 _]
      tunnel: w311 -> [w348 _]
      tunnel: w307 -> [w403 _]
      tunnel: w306 -> [w402 _]
      tunnel: [w397 w526] -> w305
      tunnel: w304 -> [w396 w526]
      tunnel: w301 -> [w357 _]
      tunnel: w300 -> [w387 w524]
      tunnel: w299 -> [w352 _]
      tunnel: w292 -> [w378 w523]
      tunnel: [w355 w523] -> w290
      tunnel: w289 -> [w362 w522]
      tunnel: w288 -> [w366 _]
      tunnel: w287 -> [w365 w521]
      tunnel: [w364 w521] -> w286
      tunnel: [w363 w522] -> w285
      tunnel: w284 -> [w359 w520]
      tunnel: [w358 w520] -> w283
      tunnel: w279 -> [w336 _]
      frame No Error {
        w405 = 12100000000000.0 ("x")
        # "Important Output"
        # "Make Sure 50Ohm"
        n148 = Increment(x=w359) -> (x+1=w360:dbl)
        n149 = case shown="False" w336 {
          tunnel: w352 -> [w441 w451]
          tunnel: w351 -> [w440 w450]
          tunnel: w350 -> [w439 w449]
          tunnel: w349 -> [_ w448]
          tunnel: w348 -> [_ w447]
          tunnel: [w438 w446] -> w347
          tunnel: [w435 w442] -> w343
          tunnel: [w435 w443] -> w342
          tunnel: [w437 w444] -> w341
          tunnel: [w436 w445] -> w340
          frame False {
            w435 = T20 {"first point time"=0.0, "xIncrement"=0.0, "Waveforms"=[]} ("Waveforms")
            # "SA"
            n150 = Index Array(array=w441, index #1=w440, index #2=w439) -> (element #1=w436:T20, element #2=w437:T20)
            n151 = Build Array(w436, w437) -> (w438:T12)
          }
          frame True {
            # "BA"
            n152 = Index Array(array=w451, index #1=w450, index #2=w449, index #3=w448, index #4=w447) -> (element #1=w445:T20, element #2=w444:T20, element #3=w443:T20, element #4=w442:T20)
            n153 = Build Array(w445, w444, w443, w442) -> (w446:T12)
          }
        }
        n154 = Add(x=w360, y=0.0) -> (x+y=w358:dbl)
        "Acquisition #" <- w358
        n155 = String To Path(string="Location") -> (path=w400:path)
        n156 = event shown="[1] \"Write Raw File?\", \"Location\": Value Change" {
          selector: _ -> [_ _]
          dyn-events: _ -> [_ _]
          timeout: 1 -> [_ _]
          tunnel: w400 -> [w477 w489]
          tunnel: [w472 w486] -> w388
          tunnel: w396 -> [w471 w485]
          tunnel: [w470 w484] -> w395
          event Timeout {
            n157 = event-data() -> ()  [unwired: 1 in, 1 out]
            n158 = local read "Write Raw File?"() -> (w469:bool)
            n159 = call <vilib>:"Check if File or Folder Exists.vi"("path"=w477) -> ("file or folder exists?"=w476:bool, "dup path"=w473:path)  [unwired: 8 in, 1 out]
            n160 = Not(x=w476) -> (.not. x?=w475:bool)
            n161 = And(x=w475, y=w469) -> (x .and. y?=w474:bool)
            n162 = case shown="True" w474 {
              tunnel: [w479 w482] -> w472
              tunnel: w473 -> [w479 w481]
              tunnel: w471 -> [w478 _]
              tunnel: [w478 0] -> w470
              frame False {
              }
              frame True {
                n163 = Create Folder(path (use dialog)=w481) -> (created path=w482:path)  [unwired: 2 in, 2 out]
              }
            }
          }
          event "Write Raw File?", "Location": Value Change {
            n164 = event-data() -> ()  [unwired: 1 in, 1 out]
            n165 = local read "Write Raw File?"() -> (w483:bool)
            n166 = call <vilib>:"Check if File or Folder Exists.vi"("path"=w489) -> ("file or folder exists?"=w488:bool, "dup path"=w487:path)  [unwired: 8 in, 1 out]
            n167 = Not(x=w488) -> (.not. x?=w491:bool)
            n168 = And(x=w491, y=w483) -> (x .and. y?=w490:bool)
            n169 = case shown="True" w490 {
              tunnel: [w493 w496] -> w486
              tunnel: w487 -> [w493 w495]
              tunnel: w485 -> [w492 _]
              tunnel: [w492 0] -> w484
              frame False {
              }
              frame True {
                n170 = Create Folder(path (use dialog)=w495) -> (created path=w496:path)  [unwired: 2 in, 2 out]
              }
            }
          }
        }
        "created path" <- w388
        n171 = Tick Count (ms)() -> (millisecond timer value=w371:u32)
        n172 = Unbundle(w340) -> ("xIncrement"=w392:dbl, "Waveforms"=w386:dbl[])  [unwired: 1 out]
        n173 = Unbundle(w341) -> ("Waveforms"=w385:dbl[])  [unwired: 2 out]
        n174 = Unbundle(w342) -> ("Waveforms"=w384:dbl[])  [unwired: 2 out]
        n175 = Unbundle(w343) -> ("Waveforms"=w383:dbl[])  [unwired: 2 out]
        n176 = Subtract(x=w371, y=w366) -> (x-y=w363:u32)
        n177 = Subtract(x=w363, y=w362) -> (x-y=w372:u32)
        n178 = Divide(x=w372, y=1000.0) -> (x/y=w370:dbl)
        "Time Between Triggers" <- w370
        n179 = Rotate 1D Array(1:w365, 2:1 ("n")) -> (0:w375:dbl[])
        n180 = Bundle By Name("t0"=w357, "Y"=w386, "dt"=w392) -> (w337:waveform(dbl))  [unwired: 1 in]
        n181 = Bundle By Name("Y"=w385, "dt"=w392) -> (w345:waveform(dbl))  [unwired: 1 in]
        n182 = Bundle By Name("Y"=w384, "dt"=w392) -> (w346:waveform(dbl))  [unwired: 1 in]
        "Charge Detector/PSU gate (CH2)" <- w346
        n183 = Bundle By Name("Y"=w383, "dt"=w392) -> (w344:waveform(dbl))  [unwired: 1 in]
        "Final Detector (CH3)" <- w344
        n184 = Array Max & Min(array=w385) -> (min index (indices)=w394:i32)  [unwired: 3 out]
        n185 = Array Max & Min(array=w386) -> (min index (indices)=w393:i32)  [unwired: 3 out]
        n186 = Replace Array Subset(array=w375, new element=w370, index=0) -> (w364:dbl[])
        n187 = case shown="False" w336 {
          tunnel: w346 -> [_ w434]
          tunnel: w345 -> [w428 w433]
          tunnel: w337 -> [w427 w432]
          tunnel: w344 -> [_ w430]
          tunnel: [w429 w431] -> w339
          tunnel: [w427 w430] -> w338
          frame False {
            # "SA"
            n188 = Build Array(w427, w428) -> (w429:waveform(dbl)[])
          }
          frame True {
            # "BA"
            n189 = Build Array(w432, w433, w434, w430) -> (w431:waveform(dbl)[])
          }
        }
        n190 = call-poly <vilib>:"Mean.vi"("X"=w364) -> ("mean"=w369:dbl)  [unwired: 1 out]
        n191 = Subtract(x=w394, y=w393) -> (x-y=w422:i32)
        n192 = Divide(x=0.6, y=w422) -> (x/y=w420:dbl)
        n193 = Build Array(w337, w345) -> (→"Velocity Detectors (CH0 & CH1)":waveform(dbl)[])
        n194 = Divide(x=w420, y=w392) -> (x/y=w418:dbl)
        n195 = Reciprocal(x=w369) -> (1/x=→"Average Frequency":dbl)
        n196 = Bundle("mean"=w369, "Ideal Time (Cursor)"="Ideal Time (Cursor)") -> (→"?":cluster{"mean":dbl, "Ideal Time (Cursor)":dbl})  [unwired: 1 in]
        n197 = Greater?(x=w418, y=0.0 ("x")) -> (0:w419:bool)
        n198 = call "Filter"("error in (no error)"=w378, "Signal"=w338) -> ("error out"=w391:errorcluster, "Filtered Signal"=w406:dynamicdata)  [unwired: 8 in]
        n199 = case shown="False" w419 {
          tunnel: w418 -> [_ w519]
          tunnel: [w518 w519] -> w380
          frame False {
            w518 = 500.0 ("Velocity")
            n200 = property on="Velocity (Est.)" class="DigNum (strict)"("Value"=w518) -> ()  [unwired: 2 in, 2 out]
          }
          frame True {
            "Velocity (Est.)" <- w519
          }
        }
        n201 = call "Convert from Dynamic Data"("Dynamic Data Type"=w406) -> ("Array"=w416:dbl[])  [unwired: 3 in]
        n202 = Array Max & Min(array=w416) -> (min value=w415:dbl)  [unwired: 3 out]
        n203 = Reciprocal(x=w405) -> (1/x=w404:dbl)
        n204 = Absolute Value(x=w415) -> (abs(x)=w414:dbl)
        n205 = Multiply(x="Acceleration Voltage (MV)", y=1000000.0) -> (x*y=w389:dbl)
        n206 = Multiply(x=w414, y=w404) -> (x*y=w381:dbl)
        "Charge" <- w381
        n207 = Multiply(x=w389, y=w381) -> (x*y=w413:dbl)
        n208 = case shown="True" "Write Raw File?" {
          tunnel: w339 -> [_ w501]
          tunnel: [w498 w515] -> w354
          tunnel: w391 -> [w500 w513]
          tunnel: w403 -> [_ w502]
          tunnel: w402 -> [w499 w511]
          tunnel: w388 -> [_ w509]
          tunnel: [w497 w507] -> w397
          tunnel: w395 -> [w497 w506]
          frame False {
            n209 = Merge Errors(w499, w500) -> (w498:errorcluster)
          }
          frame True {
            n210 = Path To String(path=w509) -> (string=w504:string)
            n211 = Format Value(format string="%05.0", value (0)=w506) -> (output string=w508:string)  [unwired: 1 in]
            n212 = Concatenate Strings(w504, "\\" ("string"), "WFM Tag", w508) -> (w517:string)
            n213 = String To Path(string=w517) -> (path=w510:path)
            n214 = Bundle(w510, w501) -> (w512:cluster{path, waveform(dbl)[]})  [unwired: 1 in]
            "output cluster" <- w512
            n215 = Merge Errors(w511, w513) -> (w514:errorcluster)
            n216 = Enqueue Element(queue=w502, element=w512, error in (no error)=w514) -> (error out=w515:errorcluster)  [unwired: 1 in, 2 out]
            n217 = Increment(x=w506) -> (x+1=w507:i32)
          }
        }
        n218 = Square(x=w380) -> (x^2=w412:dbl)
        n219 = Divide(x=w413, y=w412) -> (x/y=w382:dbl)
        "Mass" <- w382
        n220 = Build Array (concatenate)(w387, w380) -> (w409:dbl[])
        n221 = Build Array (concatenate)(w407, w382) -> (w408:dbl[])
        n222 = case shown="False" w336 {
          frame False {
            # "SA"
          }
          frame True {
            # "BA"
            n223 = shared-variable "My Computer\\Network Shared Variables.lvlib\\FPGA Trigger"(TRUE ("FPGA Trigger")) -> ()  [unwired: 1 in, 1 out]
            n224 = call "FPGA Triggered Global.vi"("Action"=Action_Items."Set", "Input"=TRUE) -> ()  [unwired: 9 in, 1 out]
          }
        }
        n225 = Bundle By Name(cluster=T13 {"Time Stamp"=timestamp(0 s since 1904-01-01), "Velocity"=0.0, "Mass"=0.0, "Charge"=0.0, "Radius"=0.0, "Array"=[], "Dust Event ID"=0, "Passed_3rd_Detector"=FALSE, "Estimate Source"=0, "Estimate Quality"=0.0} ("Input Data"), "Velocity"=w380, "Mass"=w382, "Charge"=w381) -> (w356:T13)
        n226 = Bundle "Bundle"(w409, w408) -> (→"Multi Plot 2":cluster{dbl[], dbl[]})  [unwired: 1 in]
        n227 = case shown="True" "Write to Database?" {
          tunnel: w347 -> [_ w458]
          tunnel: w357 -> [_ w457]
          tunnel: w356 -> [_ w456]
          tunnel: [w452 w455] -> w355
          tunnel: w354 -> [w452 w454]
          tunnel: w336 -> [_ w453]
          frame False {
          }
          frame True {
            n228 = case shown="False" w453 {
              tunnel: w458 -> [w459 w468]
              tunnel: w457 -> [w460 w467]
              tunnel: w456 -> [w461 w466]
              tunnel: [w462 w465] -> w455
              tunnel: w454 -> [w463 w464]
              frame False {
                n229 = call "Call_enqueue_small.vi"("Waveform"=w459, "error in"=w463, "Input Data"=w461, "seconds since 1Jan1904"=w460) -> ("error IO"=w462:errorcluster)  [unwired: 7 in]
              }
              frame True {
                n230 = call "Call_enqueue.vi"("Waveform"=w468, "error in"=w464, "Input Data"=w466, "seconds since 1Jan1904"=w467) -> ("error IO"=w465:errorcluster)  [unwired: 7 in]
              }
            }
          }
        }
        "Calibration" <- w405
      }
      frame Error {
      }
    }
    n231 = case shown="True" "Limit Triggers" {
      tunnel: [FALSE w530] -> w294
      frame False {
      }
      frame True {
        n232 = local read "Acquisition #"() -> (w529:i32)
        n233 = Decrement(x="Limit") -> (x-1=w528:dbl)
        n234 = Equal?(x=w528, y=w529) -> (x = y?=w530:bool)
      }
    }
    n235 = Or(x=w294, y="stop") -> (x .or. y?=w295:bool)
    "Stop condition" <- w295
    n236 = call <vilib>:"Clear Errors.vi"("error in (no error)"=w290) -> ("error out"=w291:errorcluster)  [unwired: 6 in]
  }
  n237 = Obtain Queue(name (unnamed)=w29, element data type=w28, error in (no error)=w27) -> (queue out=w35:refnum<queue>, error out=w34:errorcluster)  [unwired: 2 in, 1 out]
  n238 = while {
    tunnel: w35 -> [w734]
    tunnel: w34 -> [w727]
    tunnel: [w743] -> w33
    tunnel: [w741] -> w32
    i -> [w737]
    stop <- w740 stop-if-true
    n239 = local read "Stop condition"() -> (w729:bool)
    n240 = local read "Write Raw File?"() -> (w731:bool)
    n241 = Get Queue Status(queue=w734, error in (no error)=w727) -> (queue out=w728:refnum<queue>, error out=w735:errorcluster, # elements in queue=w733:i32)  [unwired: 1 in, 5 out]
    "# elements in queue" <- w733
    n242 = And(x=w731, y=w729) -> (x .and. y?=w742:bool)
    n243 = Not Equal To 0?(x=w733) -> (x != 0?=w732:bool)
    n244 = property on="Saving Raw File..." class="Path"("Blinking"=w742) -> ()  [unwired: 2 in, 2 out]
    n245 = And(x=w732, y=w731) -> (x .and. y?=w736:bool)
    n246 = local read "Stop condition"() -> (w730:bool)
    n247 = case shown="True" w736 {
      tunnel: w728 -> [w747 w766]
      tunnel: [w745 w764] -> w741
      tunnel: [w746 w762] -> w743
      tunnel: w730 -> [w748 w761]
      tunnel: [w748 w758] -> w738
      tunnel: w735 -> [w744 w754]
      frame False {
        n248 = Flush Queue(queue=w747, error in (no error)=w744) -> (queue out=w746:refnum<queue>, error out=w745:errorcluster)  [unwired: 1 out]
      }
      frame True {
        n249 = Dequeue Element(queue=w766, error in (no error)=w754) -> (queue out=w763:refnum<queue>, element=w765:cluster{path, waveform(sgl)[]}, error out=w752:errorcluster)  [unwired: 1 in, 1 out]
        n250 = Unbundle(w765) -> (w753:path, w749:waveform(sgl)[])
        n251 = Get Queue Status(queue=w763, error in (no error)=w752) -> (queue out=w762:refnum<queue>, error out=w751:errorcluster, # elements in queue=w760:i32)  [unwired: 1 in, 5 out]
        n252 = Equal To 0?(x=w760) -> (x = 0?=w759:bool)
        n253 = call <vilib>:"Check if File or Folder Exists.vi"("error in (no error)"=w751, "path"=w753) -> ("error out"=w750:errorcluster, "file or folder exists?"=w757:bool, "dup path"=w756:path)  [unwired: 7 in]
        n254 = case shown="True" w757 {
          tunnel: w756 -> [w767 _]
          tunnel: [w767 w773] -> w755
          frame False {
          }
          frame True {
            n255 = local read "created path"() -> (w770:path)
            n256 = local read "WFM Tag"() -> (w775:string)
            n257 = File/Directory Info(path=w770) -> (size=w771:i64)  [unwired: 1 in, 6 out]
            n258 = Format Value(format string="%05.0", value (0)=w771) -> (output string=w774:string)  [unwired: 1 in]
            n259 = Path To String(path=w770) -> (string=w768:string)
            n260 = Concatenate Strings(w768, "\\" ("string"), w775, w774) -> (w772:string)
            n261 = String To Path(string=w772) -> (path=w773:path)
          }
        }
        "Saving Raw File..." <- w755
        n262 = And(x=w759, y=w761) -> (x .and. y?=w758:bool)
        n263 = Write to Binary File(file (use dialog)=w755, data=w749, error in=w750) -> (error out=w764:errorcluster)  [unwired: 3 in, 2 out]
      }
    }
    n264 = Unbundle By Name(w741) -> ("status"=w739:bool)
    n265 = Or(x=w738, y=w739) -> (x .or. y?=w740:bool)
    "Numeric" <- w737
  }
  n266 = Release Queue(queue=w33, error in (no error)=w32) -> (error out=w18:errorcluster)  [unwired: 1 in, 2 out]
  n267 = call <vilib>:"Clear Errors.vi"("error in (no error)"=w18) -> ("error out"=w17:errorcluster)  [unwired: 6 in]
  n268 = Merge Errors(w17, w23, w12) -> (w19:errorcluster)
  n269 = for {
    tunnel: w38 -> [w777] mode=indexing
    shift-right: [w779] -> w50
    shift-left: w19 -> [w778]
    # "13"
    n270 = call <instrlib>:"niScope Close.vi"("instrument handle"=w777, "error in"=w778) -> ("error out"=w779:errorcluster)  [unwired: 13 in]
  }
  n271 = call <vilib>:"General Error Handler.vi"("type of dialog (OK msg:1)"=w20, "error in (no error)"=w50) -> ("message"=w46:string, "error out"=w48:errorcluster)  [unwired: 9 in, 3 out]
  n272 = Bundle By Name(cluster=w48, "source"=w46) -> (→"error out":errorcluster)
